vi "DP-Init StimGen (F1L1).vi"(0 "StimGen":T1, 1 "Expt State":T3, 5 "DP stimulus params":T4={"Start (dB)"=20.0, "Stop (dB)"=80.0, "Step (dB)"=10.0, "Ear"=enum."Left", "f2 (kHz)"="", "f1"=0.0, "f1 mode"=enum."re f2", "L1"=0.0, "L1 mode"=enum."re L2"}, 11 "error in (no error)":errorcluster, 12 "Recalibrate?":bool, 13 "Mic  gain (dB)":dbl) -> (4 "StimGen (out)":T1, 6 "DP Freqs":T2[](array[typedef]), 15 "error out":errorcluster)   [LabVIEW 2020]
uses:
  Typedefs/DP-Stim Params (F1L1).ctl
  Utility VIs/Type Defs/Left-Right ring.ctl
  CFTS Main Panel SubVIs/CFTS-Experiment State.ctl
  Typedefs/DP-Freqs.ctl
  Typedefs/DP-StimGen.ctl
  Misc VIs/Connection Manager/Type Defs/Output sources.ctl
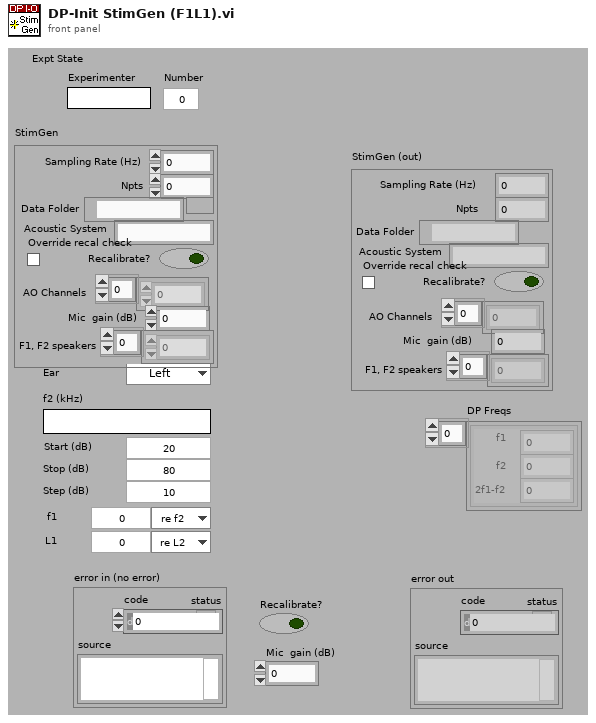
[diagram p1: front panel]
types:
  T1 = typedef "DP-StimGen.ctl" = cluster{"Sampling Rate (Hz)":dbl, "Npts":i32, "Data Folder":path, "Acoustic System":string, "Recalibrate?":bool, "AO Channels":i32[], "Mic  gain (dB)":dbl, "F1, F2 speakers":i32[], "Override recal check":bool}
  T2 = typedef "DP-Freqs.ctl" = cluster{"f1":dbl, "f2":dbl, "2f1-f2":dbl}
  T3 = typedef "CFTS-Experiment State.ctl" = cluster{"Experimenter":string, "Number":u32, "Right":string, "Left":string, "Data Folder":path, "State File":path, "Version Info":string, "End Exposure Time":dbl, "Exposure Duration":string, "Run #":cluster{"CAP":i16, "ABR":i16, "DP":i16, "VsEP":i16, "MeasSeq":i16, "SubSeq":i16, "SFOAE":i16}}
  T4 = typedef "DP-Stim Params (F1L1).ctl" = cluster{"Start (dB)":dbl, "Stop (dB)":dbl, "Step (dB)":dbl, "Ear":T5, "f2 (kHz)":string, "f1":dbl, "f1 mode":enum16{"re f2", "kHz"}, "L1":dbl, "L1 mode":enum16{"re L2", "dB"}}
  T5 = typedef "Left-Right ring.ctl" = enum16{"Right", "Left"}
  T6 = typedef "Output sources.ctl" = u16
  T7 = cluster{"Coerced Frequency (kHz)":dbl, "Coerced Frequency (kHz)":dbl, dbl}
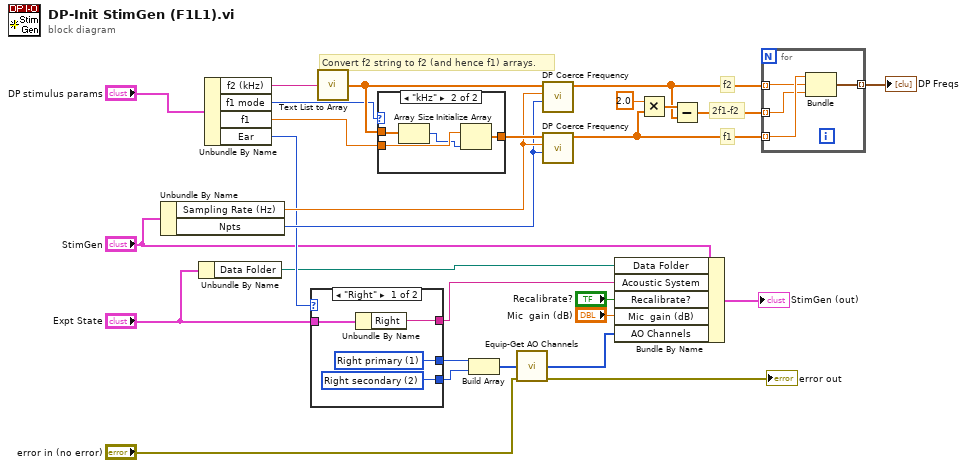
[diagram p0: block diagram]
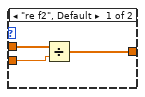
[diagram p2: hidden frame]
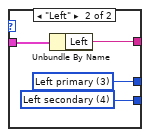
[diagram p3: hidden frame]
diagram:
  # "2f1-f2"
  # "f2"
  # "f1"
  # "Convert f2 string to f2 (and hence f1) arrays."
  n1 = Unbundle By Name("StimGen") -> ("Sampling Rate (Hz)"=w16:dbl, "Npts"=w15:i32)
  n2 = Unbundle By Name("Expt State") -> ("Data Folder"=w10:path)
  n3 = Unbundle By Name("DP stimulus params") -> ("f2 (kHz)"=w28:string, "f1 mode"=w2:enum16{"re f2", "kHz"}, "f1"=w1:dbl, "Ear"=w14:T5)
  n4 = case shown="\"Right\"" w14 {
    tunnel: [w32 w36] -> w20
    tunnel: [w31 w35] -> w19
    tunnel: "Expt State" -> [w30 w34]
    tunnel: [w29 w33] -> w5
    frame "Right" {
      w31 = T6 2 items=["--unused--", "Right primary", "Right secondary", "Left primary", "Left secondary", "Shocks", "Startle", "Background"] ("Ring")
      w32 = T6 1 items=["--unused--", "Right primary", "Right secondary", "Left primary", "Left secondary", "Shocks", "Startle", "Background"] ("Ring")
      n5 = Unbundle By Name(w30) -> ("Right"=w29:string)
    }
    frame "Left" {
      w35 = T6 4 items=["--unused--", "Right primary", "Right secondary", "Left primary", "Left secondary", "Shocks", "Startle", "Background"] ("Ring")
      w36 = T6 3 items=["--unused--", "Right primary", "Right secondary", "Left primary", "Left secondary", "Shocks", "Startle", "Background"] ("Ring")
      n6 = Unbundle By Name(w34) -> ("Left"=w33:string)
    }
  }
  n7 = call "Text List to Array.vi"("text list"=w28) -> ("array"=w27:dbl[])  [unwired: 3 in]
  n8 = case shown="\"kHz\"" w2 {
    tunnel: w27 -> [w39 w40]
    tunnel: [w38 w43] -> w26
    tunnel: w1 -> [w37 w42]
    frame "re f2", Default {
      n9 = Divide(x=w39, y=w37) -> (x/y=w38:dbl[])
    }
    frame "kHz" {
      n10 = Array Size(array=w40) -> (size(s)=w41:i32)
      n11 = Initialize Array(w42, w41) -> (w43:dbl[])
    }
  }
  n12 = Build Array(w20, w19) -> (w17:T6[])
  n13 = call "Equip-Get AO Channels.vi"("Outputs"=w17, "error in (no error)"="error in (no error)") -> ("AO Channels"=w4:i32[], "error out"=→"error out":errorcluster)  [unwired: 12 in]
  n14 = call "DP Coerce Frequency.vi"("Npts"=w15, "Sampling rate (Hz)"=w16, "Frequency (kHz)"=w27) -> ("Coerced Frequency (kHz)"=w24:dbl[])  [unwired: 6 in, 2 out]
  n15 = call "DP Coerce Frequency.vi"("Npts"=w15, "Sampling rate (Hz)"=w16, "Frequency (kHz)"=w26) -> ("Coerced Frequency (kHz)"=w22:dbl[])  [unwired: 6 in, 2 out]
  n16 = Bundle By Name(cluster="StimGen", "Data Folder"=w10, "Acoustic System"=w5, "Recalibrate?"="Recalibrate?", "Mic  gain (dB)"="Mic  gain (dB)", "AO Channels"=w4) -> (→"StimGen (out)":T1)
  n17 = Multiply(x=2.0 ("y"), y=w22) -> (x*y=w25:dbl[])
  n18 = Subtract(x=w25, y=w24) -> (x-y=w21:dbl[])
  n19 = for {
    tunnel: w24 -> [w46] mode=indexing
    tunnel: w22 -> [w47] mode=indexing
    tunnel: w21 -> [w45] mode=indexing
    tunnel: [w44] -> w8 mode=indexing
    n20 = Bundle("Coerced Frequency (kHz)"=w47, "Coerced Frequency (kHz)"=w46, w45) -> (w44:T7)  [unwired: 1 in]
  }
  "DP Freqs" <- w8
